vi "Unzip Files.vi"(8 "Error In":errorcluster, 11 "Revert Config":T1={"Revert Paths"={"Archive Path"=path "D:/workspace/revert/todo/todo.zip", "Unzip Directory"=path "D:/workspace/revert/unzip", "Backsave Directory"=path "D:/workspace/revert/backsave", "Output Archive"=path "D:/workspace/revert/backsave", "Backsave Common Directory"=path "D:/workspace/revert/backsave"}, "LabVIEW Files"={"Projects"=[], "Libraries"=[], "Classes"=[], "XControls"=[], "VIs and Controls"=[], "Non LV Files"=[]}, "LabVIEW Version"=enum."8.0"}) -> (0 "Error Out":errorcluster, 2 "Unzipped Files":path[](array[path]), 3 "Revert Config":T1={"Revert Paths"={"Archive Path"=path "D:/workspace/revert/todo/todo.zip", "Unzip Directory"=path "D:/workspace/revert/unzip", "Backsave Directory"=path "D:/workspace/revert/backsave", "Output Archive"=path "D:/workspace/revert/backsave", "Backsave Common Directory"=path "D:/workspace/revert/backsave"}, "LabVIEW Files"={"Projects"=[], "Libraries"=[], "Classes"=[], "XControls"=[], "VIs and Controls"=[], "Non LV Files"=[]}, "LabVIEW Version"=enum."8.0"})   [LabVIEW 2013, in "LVH-Revert.lvlib"]
uses:
  LVH-Revert.lvlib
  Revert Config.ctl
  Paths.ctl
  LabVIEW Files.ctl
  <vilib>/LabVIEW Hacker/LVH-Toolbox/Common/Private/Type Defs/LabVIEW Version.ctl
  <vilib>/zip/NI_Unzip.lvlib
  <vilib>/LabVIEW Hacker/LVH-Toolbox/Common/LVH-Common.lvlib
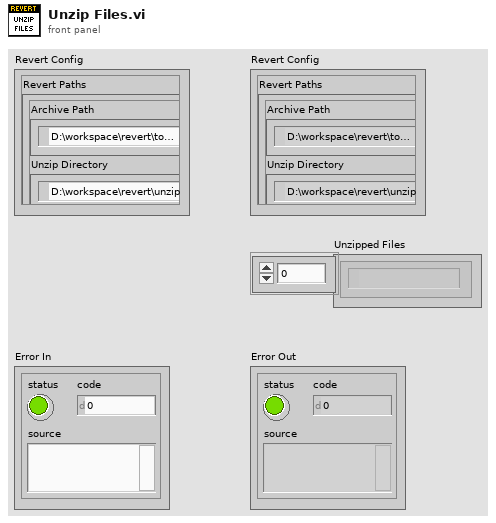
[diagram p1: front panel]
types:
  T1 = typedef "LVH-Revert.lvlib/Revert Config.ctl" = cluster{"Revert Paths":T2, "LabVIEW Files":T3, "LabVIEW Version":T4}
  T2 = typedef "LVH-Revert.lvlib/Paths.ctl" = cluster{"Archive Path":path, "Unzip Directory":path, "Backsave Directory":path, "Output Archive":path, "Backsave Common Directory":path}
  T3 = typedef "LVH-Revert.lvlib/LabVIEW Files.ctl" = cluster{"Projects":path[], "Libraries":path[], "Classes":path[], "XControls":path[], "VIs and Controls":path[], "Non LV Files":path[]}
  T4 = typedef "LVH-Toolbox.lvlib/LVH-Common.lvlib/LabVIEW Version.ctl" = enum16{"8.0", "8.2", "8.6", "9.0", "10.0", "11.0", "12.0", "13.0"}
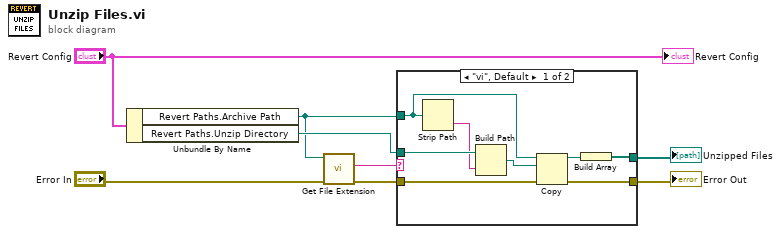
[diagram p0: block diagram]
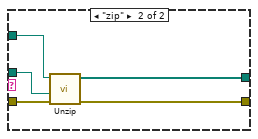
[diagram p2: hidden frame]
diagram:
  n1 = Unbundle By Name("Revert Config") -> ("Revert Paths.Archive Path"=w1:path, "Revert Paths.Unzip Directory"=w2:path)
  n2 = call <vilib>:"Get File Extension.vi"("error in (no error)"="Error In", "file"=w1) -> ("error out"=w5:errorcluster, "lowercase file extension"=w6:string)  [unwired: 6 in, 2 out]
  n3 = case shown="\"vi\", Default" w6 {
    tunnel: w5 -> [w16 w21]
    tunnel: [w15 w20] -> w4
    tunnel: [w9 w19] -> w3
    tunnel: w1 -> [w11 w18]
    tunnel: w2 -> [w14 w17]
    frame "vi", Default {
      n4 = Strip Path(path=w11) -> (name=w13:string)  [unwired: 1 out]
      n5 = Build Path(base path=w14, name or relative path=w13) -> (appended path=w12:path)
      n6 = Copy(8:w16, 10:w12, 11:w11) -> (0:w15:errorcluster, 3:w10:path)  [unwired: 2 in, 1 out]
      n7 = Build Array(w10) -> (w9:path[])
    }
    frame "zip" {
      n8 = call <vilib>:"Unzip.vi"("error in (no error)"=w21, "Target directory (same as Zip file if empty)"=w17, "Zip file"=w18) -> ("error out"=w20:errorcluster, "Unzipped files"=w19:path[])  [unwired: 6 in, 1 out]
    }
  }
  "Error Out" <- w4
  "Unzipped Files" <- w3
  "Revert Config" <- "Revert Config"
